vi "From Msgpack.vi"(4 "Byte Array as Blobs":bool=TRUE, 6 "LabPack Shared Library":path=path "", 7 "Types and Defaults":variant=variant(u8[] []), 8 "Error In":errorcluster, 11 "Msgpack Data":u8[](array[numeric])=[196, 4, 84, 101, 115, 116]) -> (0 "Error Out":errorcluster, 3 "Value":variant=variant(variant[] []))   [LabVIEW 2019, in "LabPack.lvlib"]
doc: "Converts MessagePack binary data to Variant. The <b>Type and Defaults</b> control must be provided as schema-less decoding of MessagePack data is not supported. If a cluster is used, then all elements must have labels. Each element in a cluster is decoded as a map (key-value pair), where the element's label is the key. By default, the MessagePack binary type is converted to a byte array."
uses:
  LabPack.lvlib
  Reader/Private/Begin by Value.vi
  Reader/Private/End by Value.vi
  Reader/Reader.lvclass
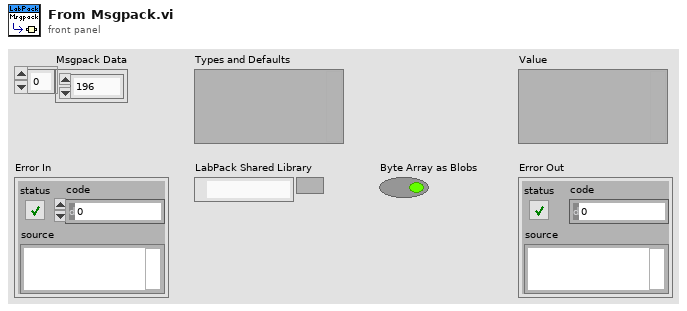
[diagram p1: front panel]
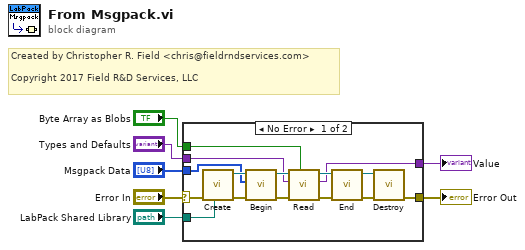
[diagram p0: block diagram]
diagram:
  # "Created by Christopher R. Field <chris@fieldrndservices.com>\n\nCopyright 2017 Field R&D Services, LLC"
  n1 = case shown="No Error" "Error In" {
    selector: "Error In" -> [w22 w23]
    tunnel: "LabPack Shared Library" -> [w9 _]
    tunnel: [w21 w23] -> w5
    tunnel: "Msgpack Data" -> [w18 _]
    tunnel: "Types and Defaults" -> [w11 _]
    tunnel: [w10 _] -> w2
    tunnel: "Byte Array as Blobs" -> [w8 _]
    frame No Error {
      n2 = call "Create.vi"("LabPack Shared Library"=w9, "Error In"=w22) -> ("Error Out"=w19:errorcluster, "Reader"=w20:refnum<class "Reader.lvclass">)  [unwired: 8 in]
      n3 = call-poly "Begin.vi"("Error In"=w19, "Msgpack Data"=w18, "Reader In"=w20) -> ("Error Out"=w12:errorcluster, "Reader Out"=w15:refnum<class "Reader.lvclass">)  [unwired: 7 in]
      n4 = call "Read.vi"("Byte Array as Blobs"=w8, "Error In"=w12, "Types and Defaults"=w11, "Reader In"=w15) -> ("Error Out"=w13:errorcluster, "Value"=w10:variant, "Reader Out"=w14:refnum<class "Reader.lvclass">)  [unwired: 5 in]
      n5 = call-poly "End.vi"("Error In"=w13, "Reader In"=w14) -> ("Error Out"=w16:errorcluster, "Reader Out"=w17:refnum<class "Reader.lvclass">)  [unwired: 8 in]
      n6 = call "Destroy.vi"("Error In"=w16, "Reader"=w17) -> ("Error Out"=w21:errorcluster)  [unwired: 9 in]
    }
    frame Error {
    }
  }
  "Error Out" <- w5
  "Value" <- w2
